vi "17.1.3 Classifier Training-Binary.vi"() -> ()   [LabVIEW 2017]
uses:
  <vilib>/vision/Classification.llb/IMAQ Classifier Nearest Neighbor Training Results.ctl
  <vilib>/vision/Classification.llb/IMAQ Classification Particle Classification options.ctl
  <vilib>/vision/Classification.llb/IMAQ Classifier Nearest Neighbor options.ctl
  <vilib>/vision/Classification.llb/IMAQ Classifier Write Options.ctl
  <vilib>/vision/NI_Vision_Development_Module.lvlib
panel:
  out "Class Distance Table":dbl[][](array[numeric]) format="%.2f"
  out "Training Results":T1[](array[typedef]) {"Standard Deviation" format="%.2f"}
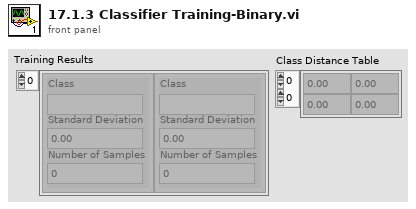
[diagram p1: front panel]
types:
  T1 = typedef "IMAQ Classifier Nearest Neighbor Training Results.ctl" = cluster{"Class":string, "Standard Deviation":sgl, "Number of Samples":i32}
  T2 = typedef "IMAQ Classifier Write Options.ctl" = i32
  T3 = typedef "IMAQ Classifier Nearest Neighbor options.ctl" = cluster{"Method":i32, "Metric":i32, "k":i32}
  T4 = typedef "IMAQ Classification Particle Classification options.ctl" = cluster{"Scale Dependence":sgl, "Mirror Dependence":sgl}
  T5 = typedef "IMAQ Classifier Session.ctl" = refnum<k1>
  T6 = typedef "IMAQ Image.ctl" = refnum<image>
  T7 = typedef "ROI Descriptor" = cluster{"Global Rectangle":i32[], "Contours":cluster{"ID":enum32{"External", "Internal"}, "Type":u32, "Coordinates":i32[]}[]}
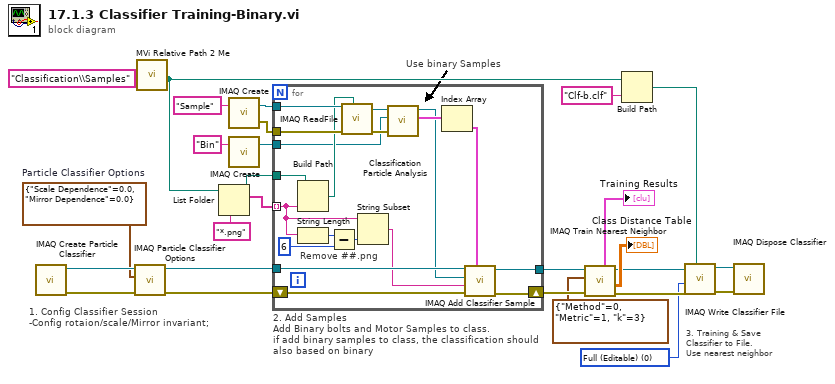
[diagram p0: block diagram]
diagram:
  w5 = T2 0 items=["Full (Editable)", "Compact (Not Editable)"] ("Write Options")
  w19 = T4 {"Scale Dependence"=0.0, "Mirror Dependence"=0.0}  # Particle Classifier Options
  # "Use binary Samples"
  # "3. Training & Save Classifier to File.\nUse nearest neighbor"
  # "2. Add Samples\nAdd Binary bolts and Motor Samples to class.\nif add binary samples to class, the classification should also based on binary"
  # "1. Config Classifier Session\n-Config rotaion/scale/Mirror invariant;"
  n1 = call "IMAQ Create Particle Classifier"() -> ("error out"=w20:errorcluster, "Classifier Session"=w21:T5)  [unwired: 10 in]
  n2 = call "IMAQ Particle Classifier Options"("error in (no error)"=w20, "Particle Classifier Options"=w19, "Classifier Session"=w21) -> ("error out"=w1:errorcluster, "Classifier Session (dup)"=w2:T5)  [unwired: 6 in, 1 out]
  n3 = call "MVi Relative Path 2 Me.vi"("Relative Path"="Classification\\Samples") -> ("Appended Dir"=w10:path)  [unwired: 5 in, 1 out]
  n4 = List Folder(path=w10, pattern="*.png") -> (path out=w22:path, filenames=w25:string[])  [unwired: 2 in, 2 out]
  n5 = call "IMAQ Create"("Image Name"="Sample") -> ("New Image"=w23:T6, "error out"=w11:errorcluster)  [unwired: 4 in]
  n6 = call "IMAQ Create"("Image Name"="Bin") -> ("New Image"=w3:T6)  [unwired: 4 in, 1 out]
  n7 = for {
    tunnel: w25 -> [w40] mode=indexing
    tunnel: w2 -> [w43]
    tunnel: w23 -> [w39]
    tunnel: w22 -> [w41]
    shift-right: [w37] -> w17
    shift-left: w1 -> [w38]
    tunnel: [w36] -> w18
    tunnel: w11 -> [w35]
    tunnel: w3 -> [w31]
    # "Remove ##.png"
    n8 = Build Path(base path=w41, name or relative path=w40) -> (appended path=w34:path)
    n9 = String Length(string=w40) -> (length=w46:i32)
    n10 = Subtract(x=w46, y=6) -> (x-y=w44:i32)
    n11 = call "IMAQ ReadFile"("File Path"=w34, "error in (no error)"=w35, "Image"=w39) -> ("error out"=w33:errorcluster, "Image Out"=w29:T6)  [unwired: 4 in, 3 out]
    n12 = String Subset(string=w40, length (rest)=w44) -> (substring=w42:string)  [unwired: 1 in]
    n13 = call "Classification Particle Analysis.vi"("error in (no error)"=w33, "Image Dest"=w31, "Image Source"=w29) -> ("ROIs"=w32:T7[], "Image Out"=w28:T6)  [unwired: 5 in, 2 out]
    n14 = Index Array(array=w32) -> (element=w30:T7)  [unwired: 1 in]
    n15 = call "IMAQ Add Classifier Sample"("ROI Descriptor"=w30, "error in (no error)"=w38, "Class"=w42, "Image"=w28, "Classifier Session"=w43) -> ("error out"=w37:errorcluster, "Classifier Session (dup)"=w36:T5)  [unwired: 4 in, 1 out]
  }
  n16 = call "IMAQ Train Nearest Neighbor"("error in (no error)"=w17, "Nearest Neighbor Options"=T3 {"Method"=0, "Metric"=1, "k"=3}, "Classifier Session"=w18) -> ("error out"=w12:errorcluster, "Class Distance Table"=→"Class Distance Table":dbl[][], "Classifier Session (dup)"=w13:T5, "Training Results"=→"Training Results":T1[])  [unwired: 5 in]
  n17 = Build Path(base path=w10, name or relative path="Clf-b.clf" ("pattern")) -> (appended path=w8:path)
  n18 = call "IMAQ Write Classifier File"("File Path"=w8, "error in (no error)"=w12, "Write Options"=w5, "Classifier Session"=w13) -> ("error out"=w7:errorcluster, "Classifier Session (dup)"=w6:T5)  [unwired: 6 in]
  n19 = call "IMAQ Dispose Classifier"("error in (no error)"=w7, "Classifier Session"=w6) -> ()  [unwired: 9 in, 1 out]
